vi "set_speeds.vi"(1 "speed rotation":u32=100000000, 2 "frequency rotation":u32=18000, 3 "error in (no error)":errorcluster, 4 "speed xy":u32=1000000, 5 "frequency xy":u32=12000) -> (0 "error out":errorcluster)   [LabVIEW 2016]
uses:
  sa commands.ctl
panel:
  out "System Index":u32=35
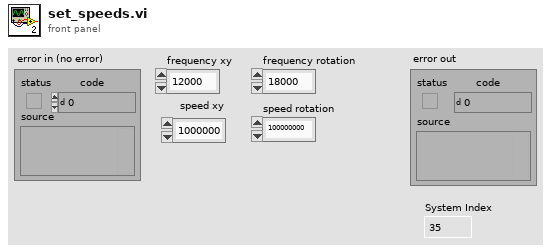
[diagram p1: front panel]
types:
  T1 = typedef "sa commands.ctl" = enum16{"read all", "set system index", "set x channel", "set y channel", "set rotation channel"}
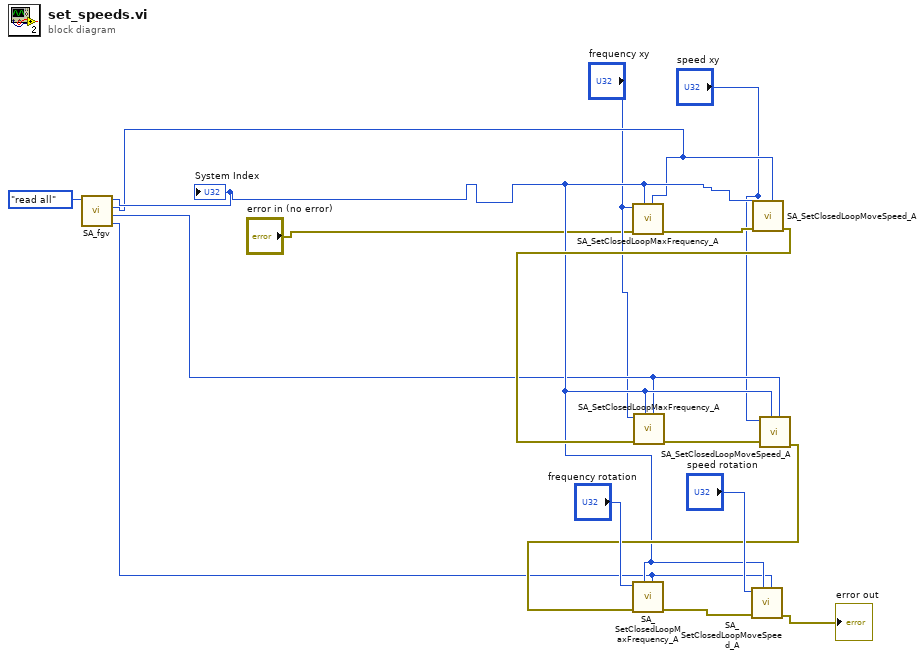
[diagram p0: block diagram]
diagram:
  n1 = call "SA_fgv.vi"("command"=sa_commands."read all") -> ("rotation channel"=w4:u32, "y channel"=w6:u32, "x channel"=w7:u32, "system index"=w8:u32)  [unwired: 3 in]
  "System Index" <- w8
  n2 = call <vilib>:"SA_SetClosedLoopMaxFrequency_A.vi"("channelIndex"=w7, "systemIndex"=w8, "error in (no error)"="error in (no error)", "frequency"="frequency xy") -> ("error out"=w14:errorcluster)  [unwired: 7 in]
  n3 = call <vilib>:"SA_SetClosedLoopMoveSpeed_A.vi"("channelIndex"=w7, "systemIndex"=w8, "error in (no error)"=w14, "speed"="speed xy") -> ("error out"=w11:errorcluster)  [unwired: 7 in]
  n4 = call <vilib>:"SA_SetClosedLoopMaxFrequency_A.vi"("channelIndex"=w6, "systemIndex"=w8, "error in (no error)"=w11, "frequency"="frequency xy") -> ("error out"=w15:errorcluster)  [unwired: 7 in]
  n5 = call <vilib>:"SA_SetClosedLoopMoveSpeed_A.vi"("channelIndex"=w6, "systemIndex"=w8, "error in (no error)"=w15, "speed"="speed xy") -> ("error out"=w10:errorcluster)  [unwired: 7 in]
  n6 = call <vilib>:"SA_SetClosedLoopMaxFrequency_A.vi"("channelIndex"=w4, "systemIndex"=w8, "error in (no error)"=w10, "frequency"="frequency rotation") -> ("error out"=w16:errorcluster)  [unwired: 7 in]
  n7 = call <vilib>:"SA_SetClosedLoopMoveSpeed_A.vi"("channelIndex"=w4, "systemIndex"=w8, "error in (no error)"=w16, "speed"="speed rotation") -> ("error out"=→"error out":errorcluster)  [unwired: 7 in]
